vi "c Spark Set CAN Max Retries.vi"(8 "error in (no error)":errorcluster, 10 "numRetries":i32, 11 "handle":T1) -> (0 "error out":errorcluster, 3 "handle out":T1)   [LabVIEW 2023, in "REVLibDriver.lvlib"]
doc: "void c_Spark_SetCANMaxRetries(c_Spark_handle handle, int numRetries);"
uses:
  REVLibDriver.lvlib
  REVLibDriver.dll
  <vilib>/Custom Controls/c_Spark_handle.ctl
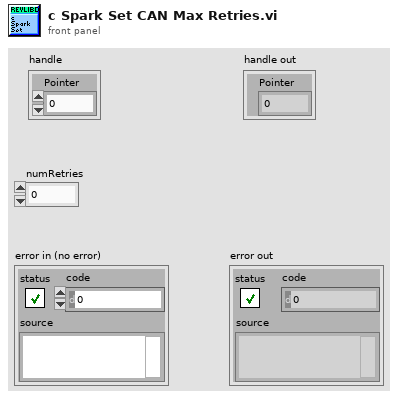
[diagram p1: front panel]
types:
  T1 = typedef "REVLibDriver.lvlib/c_Spark_handle.ctl" = cluster{"Pointer":u32}
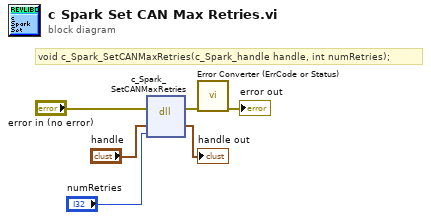
[diagram p0: block diagram]
diagram:
  # "void c_Spark_SetCANMaxRetries(c_Spark_handle handle, int numRetries);"
  n1 = dll-call lib="REVLibDriver.*" fn="c_Spark_SetCANMaxRetries"(error in="error in (no error)", "handle"="handle", "numRetries"="numRetries") -> (error out=w2:errorcluster, "handle"=→"handle out":T1)  [unwired: 4 in, 1 out]
  n2 = call "Error Converter (ErrCode or Status).vi"("error in (no error)"=w2) -> ("error out"=→"error out":errorcluster)  [unwired: 10 in]
